vi "Calc_Actuators_Length and Angle.vi"(3 "Vpot_Left":dbl=0.06 format="%.4f", 4 "Vpot_Right":dbl=0.14 format="%.4f", 7 "Actuator Cal Params":T1={"Vmax_Left"=0.5, "Vmin_Left"=0.06, "Vmax_Right"=0.53, "Vmin_Right"=0.14, "Elev_max"=50.0, "Elev_min"=-13.7} {"Elev_min" format="%.1f"; "Elev_max" format="%.1f"; "Vmin_Right" format="%.4f"; "Vmax_Right" format="%.4f"; "Vmin_Left" format="%.4f"; "Vmax_Left" format="%.4f"}) -> (13 "% Length_Avg":dbl format="%.4f", 14 "Elev Angle":dbl=-13.7 format="%.1f", 17 "% Length_Left":dbl format="%.4f", 18 "% Length_Right":dbl format="%.4f")   [LabVIEW 2017]
uses:
  Type Definitions/typedef_cluster_Actuator Calibrations.ctl
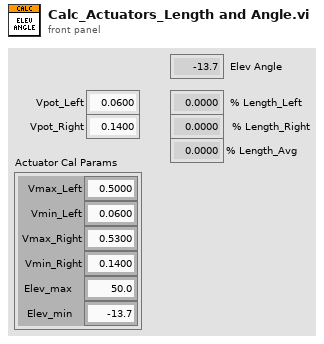
[diagram p1: front panel]
types:
  T1 = typedef "typedef_cluster_Actuator Calibrations.ctl" = cluster{"Vmax_Left":dbl, "Vmin_Left":dbl, "Vmax_Right":dbl, "Vmin_Right":dbl, "Elev_max":dbl, "Elev_min":dbl}
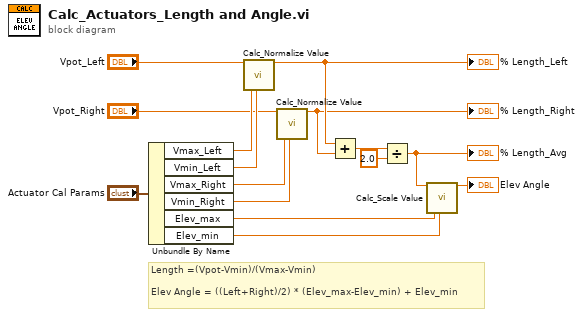
[diagram p0: block diagram]
diagram:
  # "Length =(Vpot-Vmin)/(Vmax-Vmin)\n\nElev Angle = ((Left+Right)/2) * (Elev_max-Elev_min) + Elev_min"
  n1 = Unbundle By Name("Actuator Cal Params") -> ("Vmax_Left"=w13:dbl, "Vmin_Left"=w12:dbl, "Vmax_Right"=w2:dbl, "Vmin_Right"=w1:dbl, "Elev_max"=w7:dbl, "Elev_min"=w6:dbl)
  n2 = call "Calc_Normalize Value.vi"("Value"="Vpot_Left", "Max"=w13, "Min"=w12) -> ("Normalized Value"=w10:dbl)  [unwired: 16 in]
  "% Length_Left" <- w10
  n3 = call "Calc_Normalize Value.vi"("Value"="Vpot_Right", "Max"=w2, "Min"=w1) -> ("Normalized Value"=w3:dbl)  [unwired: 16 in]
  "% Length_Right" <- w3
  n4 = Add(x=w10, y=w3) -> (x+y=w11:dbl)
  n5 = Divide(x=w11, y=2.0) -> (x/y=w8:dbl)
  "% Length_Avg" <- w8
  n6 = call "Calc_Scale Value.vi"("Normalized Value"=w8, "Max"=w7, "Min"=w6) -> ("Value"=→"Elev Angle":dbl)  [unwired: 16 in]
